vi "State machine process.vi"() -> ()   [LabVIEW 2025]
panel:
  out "Prcoess":enum16{"start", "proc 1", "stop"}(ring)
  in  "stop":bool
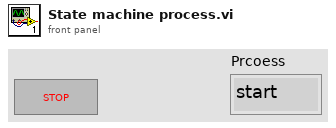
[diagram p1: front panel]
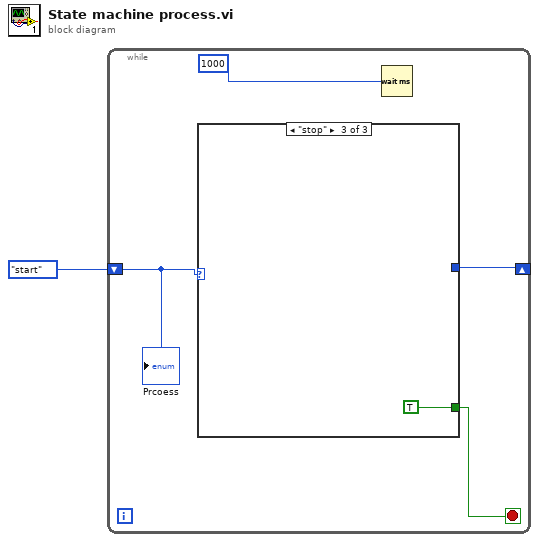
[diagram p0: block diagram]
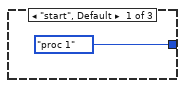
[diagram p2: hidden frame]
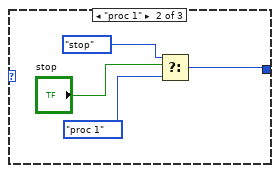
[diagram p3: hidden frame]
diagram:
  n1 = while {
    shift-right: [w5] -> _
    shift-left: enum16{"start", "proc 1", "stop"}."start" -> [w3]
    stop <- w4 stop-if-true
    n2 = case shown="\"stop\"" w3 {
      tunnel: [enum16{"start", "proc 1", "stop"}."proc 1" w7 _] -> w5
      tunnel: [_ _ TRUE] -> w4
      frame "start", Default {
      }
      frame "proc 1" {
        n3 = Select(t=enum16{"start", "proc 1", "stop"}."stop", s="stop", f=enum16{"start", "proc 1", "stop"}."proc 1") -> (s? t:f=w7:enum16{"start", "proc 1", "stop"})
      }
      frame "stop" {
      }
    }
    n4 = Wait (ms)(milliseconds to wait=u32 1000) -> ()  [unwired: 1 out]
    "Prcoess" <- w3
  }
